vi "ChoosePath.vi"(10 "Limelight Raw Horizontal Offset to Ball (deg)":dbl) -> (2 "Auto Path Suffix":string)   [LabVIEW 2020]
doc: "This VI uses LimeLight targeting data to determine the mots likely ball configuration for the 2021 Galactic Search Challenge. Once the ball configuration is known, the appropriate suffix is applied to the autonomous path name."
uses:
  sensordata.vi
panel:
  in  "Loops to Average":i32=10
  in  "Lower Bound on Blue A":dbl=-30.0
  in  "Division between Blue B and Blue A":dbl=-22.0
  in  "Division between Red A and Blue B":dbl=-13.0
  in  "Division between Red A and Red B":dbl=-5.0
  in  "Upper Bound for Red B":dbl=30.0
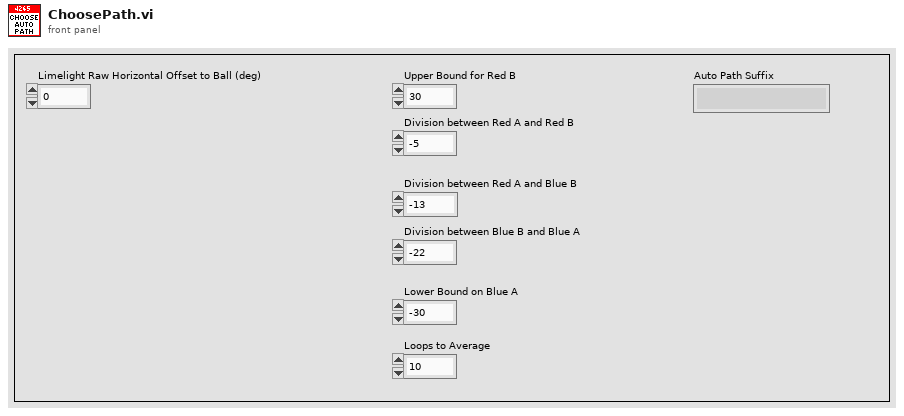
[diagram p1: front panel]
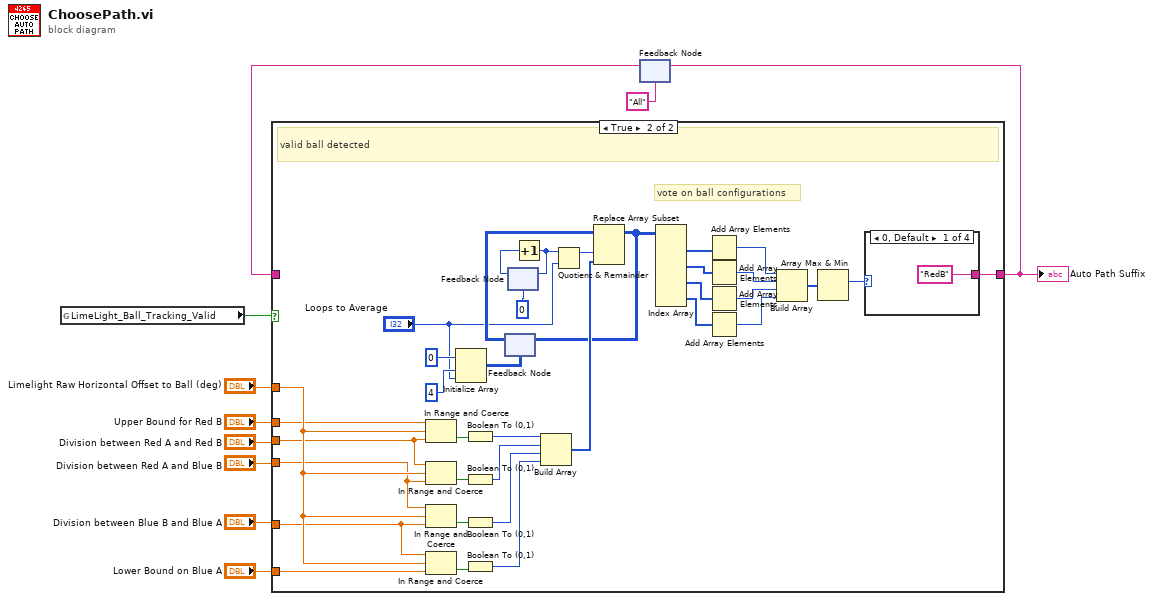
[diagram p0: block diagram]
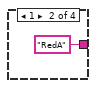
[diagram p3: hidden frame]
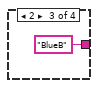
[diagram p4: hidden frame]
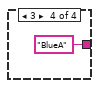
[diagram p5: hidden frame]
diagram:
  n1 = global read "sensordata.vi" "LimeLight_Ball_Tracking_Valid"() -> (w4:bool)
  n2 = feedback #1("All") -> (w1:string)
  n3 = case shown="True" w4 {
    tunnel: "Limelight Raw Horizontal Offset to Ball (deg)" -> [_ w47]
    tunnel: "Upper Bound for Red B" -> [_ w46]
    tunnel: "Division between Red A and Red B" -> [_ w45]
    tunnel: "Division between Red A and Blue B" -> [_ w44]
    tunnel: "Division between Blue B and Blue A" -> [_ w43]
    tunnel: "Lower Bound on Blue A" -> [_ w42]
    tunnel: [w11 w12] -> w2
    tunnel: w1 -> [w11 _]
    frame False {
      # "no valid ball detected"
    }
    frame True {
      # "vote on ball configurations"
      # "valid ball detected"
      n4 = In Range and Coerce(upper limit=w46, x=w47, lower limit=w45) -> (In Range?=w35:bool)  [unwired: 1 out]
      n5 = In Range and Coerce(upper limit=w45, x=w47, lower limit=w44) -> (In Range?=w33:bool)  [unwired: 1 out]
      n6 = In Range and Coerce(upper limit=w44, x=w47, lower limit=w43) -> (In Range?=w31:bool)  [unwired: 1 out]
      n7 = In Range and Coerce(upper limit=w43, x=w47, lower limit=w42) -> (In Range?=w29:bool)  [unwired: 1 out]
      n8 = Initialize Array(i16 0, 4 ("dimension size"), "Loops to Average") -> (w39:i16[][])
      n9 = Boolean To (0,1)(Boolean=w35) -> (0, 1=w34:i16)
      n10 = Boolean To (0,1)(Boolean=w33) -> (0, 1=w32:i16)
      n11 = Boolean To (0,1)(Boolean=w31) -> (0, 1=w30:i16)
      n12 = Boolean To (0,1)(Boolean=w29) -> (0, 1=w28:i16)
      n13 = feedback #2(w39) -> (w38:i16[][])
      n14 = feedback #3(0) -> (w36:i32)
      n15 = Increment(x=w36) -> (x+1=w26:i32)
      n16 = feedback-in #3(w26) -> ()
      n17 = Build Array(w34, w32, w30, w28) -> (w27:i16[])
      n18 = Quotient & Remainder(x=w26, y="Loops to Average") -> (x-y*floor(x/y)=w13:i32)  [unwired: 1 out]
      n19 = Replace Array Subset(array=w38, new element=w27, index (col)=w13) -> (w25:i16[][])  [unwired: 1 in]
      n20 = feedback-in #2(w25) -> ()
      n21 = Index Array(array=w25) -> (element #1=w24:i16[], element #2=w23:i16[], element #3=w22:i16[], element #4=w21:i16[])  [unwired: 8 in]
      n22 = Add Array Elements(numeric array=w24) -> (sum=w20:i16)
      n23 = Add Array Elements(numeric array=w23) -> (sum=w19:i16)
      n24 = Add Array Elements(numeric array=w22) -> (sum=w18:i16)
      n25 = Add Array Elements(numeric array=w21) -> (sum=w17:i16)
      n26 = Build Array(w20, w19, w18, w17) -> (w16:i16[])
      n27 = Array Max & Min(array=w16) -> (max index (indices)=w15:i32)  [unwired: 3 out]
      n28 = case shown="0, Default" w15 {
        tunnel: ["RedB" "RedA" "BlueB" "BlueA"] -> w12
        frame 0, Default {
        }
        frame 1 {
        }
        frame 2 {
        }
        frame 3 {
        }
      }
    }
  }
  "Auto Path Suffix" <- w2
  n29 = feedback-in #1(w2) -> ()
